vi "Redimesionare&Conversie.vi"(11 "Path":path) -> (0 "Image 28x28":dbl[][](array[numeric]), 1 "Nr inputs":dbl, 2 "Dimenstiune imagine":dbl[](array[numeric]), 3 "Image 1D array":dbl[](array[numeric]))   [LabVIEW 2024]
uses:
  <vilib>/vision/NI_Vision_Development_Module.lvlib
panel:
  out "Image":T1(plugin-control)
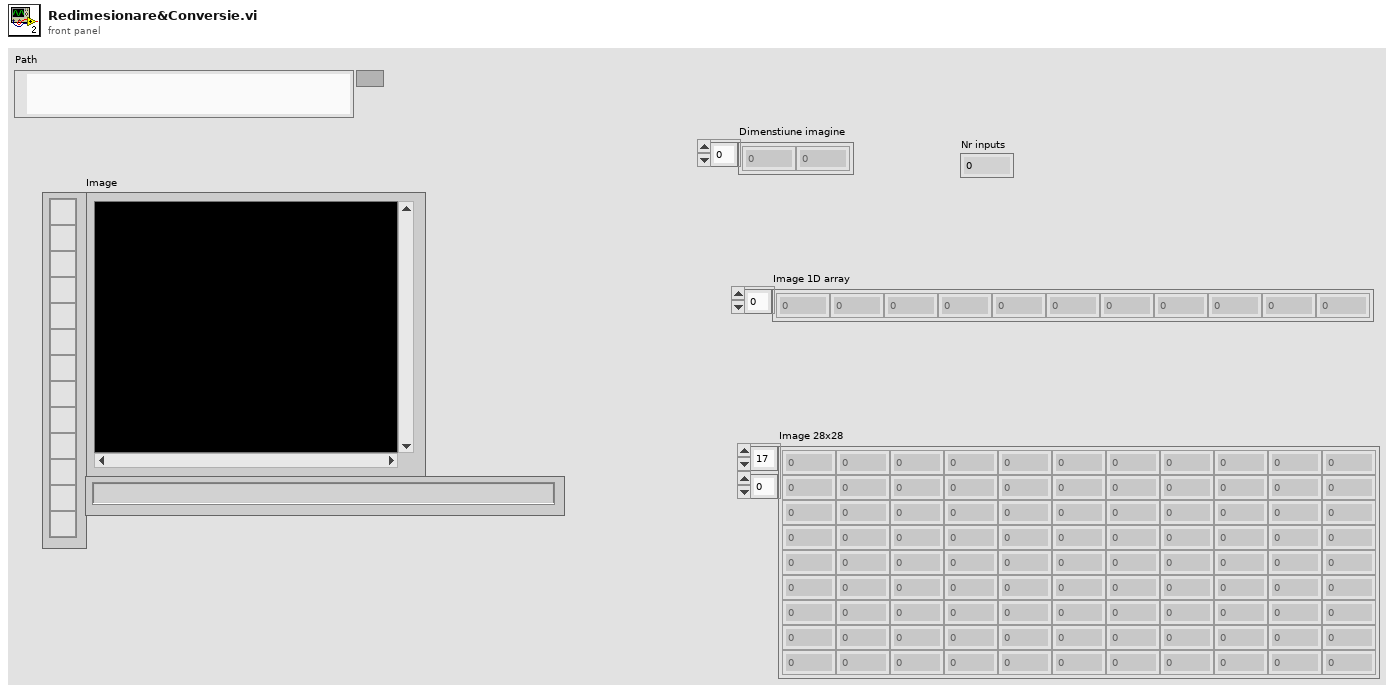
[diagram p1: front panel]
types:
  T1 = typedef "IMAQ Image.ctl" = refnum<image>
  T2 = typedef "Image Type" = u32
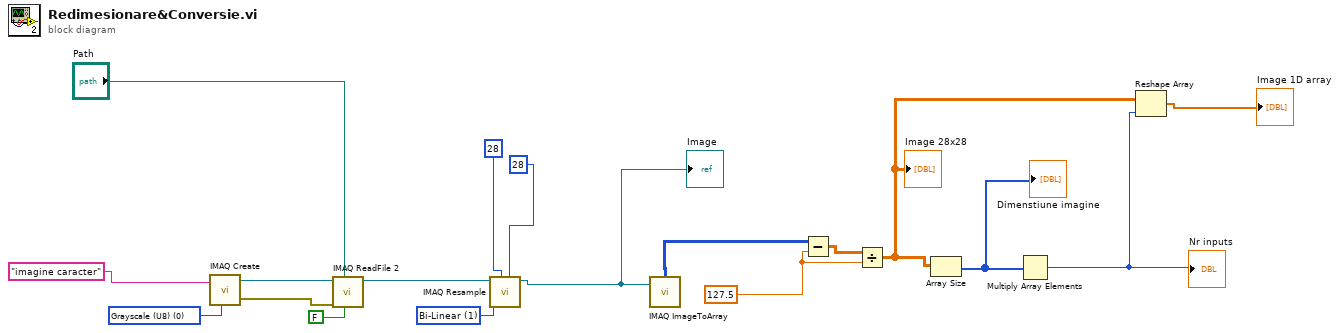
[diagram p0: block diagram]
diagram:
  w6 = 127.5
  w8 = u32 1 items=["Zero Order", "Bi-Linear", "Quadratic", "Cubic Spline"] ("Interpolation Type")
  w18 = T2 0 items=["Grayscale (U8)", "Grayscale (I16)", "Grayscale (SGL)", "Complex (CSG)", "RGB (U32)", "HSL (U32)", "RGB (U64)", "Grayscale (U16)"] ("Image Type")
  n1 = call "IMAQ Create"("Image Name"="imagine caracter", "Image Type"=w18) -> ("New Image"=w16:T1, "error out"=w17:errorcluster)  [unwired: 3 in]
  n2 = call "IMAQ ReadFile 2"("Use File Path Image Type"=FALSE, "File Path"="Path", "error in (no error)"=w17, "Image"=w16) -> ("Image Out"=w12:T1)  [unwired: 3 in, 4 out]
  n3 = call "IMAQ Resample"("X Resolution"=28, "Y Resolution"=28, "Interpolation Type"=w8, "Image Src"=w12) -> ("Image Dst Out"=w9:T1)  [unwired: 6 in, 1 out]
  "Image" <- w9
  n4 = call "IMAQ ImageToArray"("Image"=w9) -> ("Image Pixels (U8)"=w5:u8[][])  [unwired: 3 in, 4 out]
  n5 = Subtract(x=w5, y=w6) -> (x-y=w7:dbl[][])
  n6 = Divide(x=w7, y=w6) -> (x/y=w2:dbl[][])
  "Image 28x28" <- w2
  n7 = Array Size(array=w2) -> (size(s)=w4:i32[])
  "Dimenstiune imagine" <- w4
  n8 = Multiply Array Elements(1:w4) -> (0:w3:i32)
  "Nr inputs" <- w3
  n9 = Reshape Array(w2, w3) -> (→"Image 1D array":dbl[])
